vi "number2-selection sort.vi"(3 "Boolean":bool=TRUE, 4 "Array":dbl[](array[numeric]), 5 "Wait":u32=10) -> (1 "Waveform Graph":dbl[](graph))   [LabVIEW 2014]
doc: "This VI implements selection sort fully programmed in LabVIEW. In addition, it allows you to set a wait in the main loop and displays the partially sorted array so that you can see the actual process that selection sort takes to sort the array. See the Wikipedia entry for the detailed process on how the sorting is accomplished."
panel:
  in  "Number of Elements":i32=1024
  out "Max Index":u32
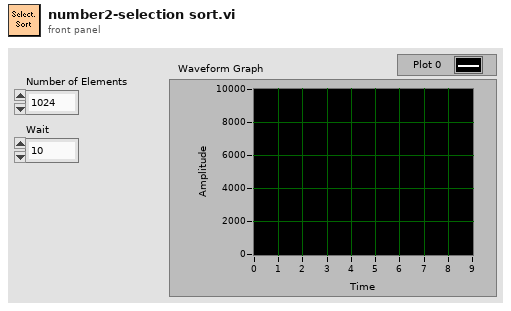
[diagram p1: front panel]
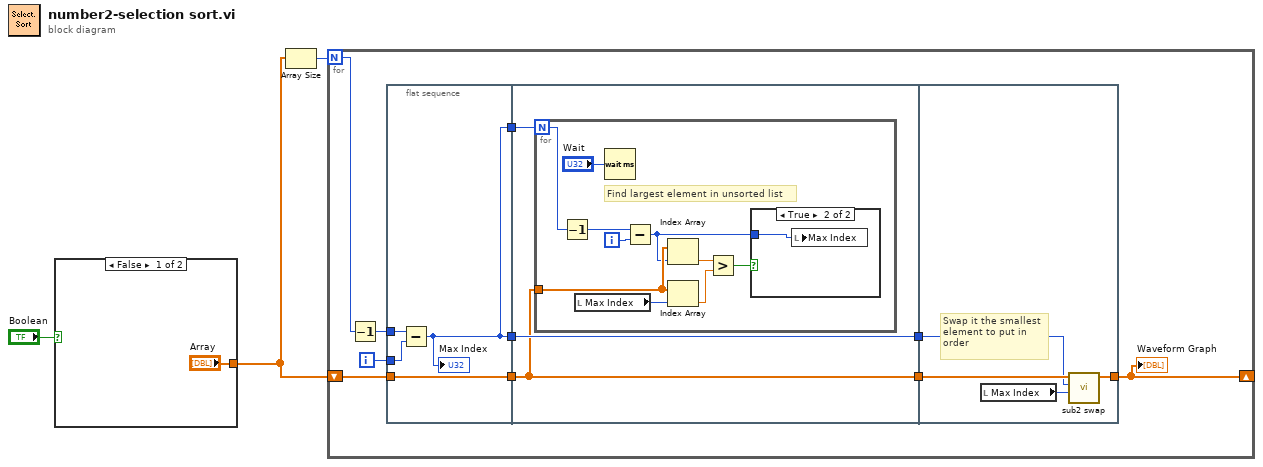
[diagram p0: block diagram]
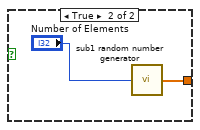
[diagram p2: hidden frame]
diagram:
  n1 = case shown="False" "Boolean" {
    tunnel: ["Array" w6] -> w1
    frame False {
    }
    frame True {
      n2 = call "sub1 random number generator.vi"("Numeric"="Number of Elements") -> ("Array"=w6:dbl[])  [unwired: 4 in]
    }
  }
  n3 = Array Size(array=w1) -> (size(s)=w3:i32)
  n4 = for {
    N: w3 -> [w10]
    shift-right: [w11] -> _
    shift-left: w1 -> [w16]
    i -> [w7]
    n5 = Decrement(x=w10) -> (x-1=w8:i32)
    n6 = flat-sequence {
      tunnel: w16 -> [w20]
      tunnel: [w20] -> w15
      tunnel: [w17] -> w12
      tunnel: [w17] -> w9
      tunnel: w8 -> [w19]
      tunnel: w7 -> [w18]
      tunnel: w15 -> [w22]
      tunnel: [w22] -> w14
      tunnel: [w23] -> w13
      tunnel: w12 -> [w23]
      tunnel: w9 -> [w21]
      tunnel: w14 -> [w38]
      tunnel: w13 -> [w37]
      tunnel: [w35] -> w11
      frame #0 {
        n7 = Subtract(x=w19, y=w18) -> (x-y=w17:i32)
        "Max Index" <- w17
      }
      frame #1 {
        n8 = for {
          N: w21 -> [w27]
          tunnel: w22 -> [w28]
          i -> [w25]
          # "Find largest element in unsorted list"
          n9 = Decrement(x=w27) -> (x-1=w26:i32)
          n10 = local read "Max Index"() -> (w33:u32)
          n11 = Wait (ms)(milliseconds to wait="Wait") -> ()  [unwired: 1 out]
          n12 = Subtract(x=w26, y=w25) -> (x-y=w24:i32)
          n13 = Index Array(array=w28, index=w24) -> (element=w32:dbl)
          n14 = Index Array(array=w28, index=w33) -> (element=w31:dbl)
          n15 = Greater?(x=w32, y=w31) -> (0:w30:bool)
          n16 = case shown="True" w30 {
            tunnel: w24 -> [_ w34]
            frame False {
            }
            frame True {
              n17 = local write "Max Index"(w34) -> ()
            }
          }
        }
      }
      frame #2 {
        # "Swap it the smallest\nelement to put in\norder"
        n18 = local read "Max Index"() -> (w36:u32)
        n19 = call "sub2 swap.vi"("Y"=w36, "X"=w37, "Original"=w38) -> ("After Swapped"=w35:dbl[])  [unwired: 4 in]
      }
    }
    "Waveform Graph" <- w11
  }
